vi "EnFlo_Data_Sync_Manual.vi"() -> ()   [LabVIEW 2012]
uses:
  Anemometry Sub Vis/Controls/EnFlo_Data_Folder_Setup.ctl
  Anemometry Sub Vis/Globals/Preference_global.vi
  Anemometry Sub Vis/Globals/Constants_global.vi
panel:
  out "error out":errorcluster
  out "Folder contents changed?":bool
  in  "Folder to Sync (Must be within Local EnFlo Data)":path=path "C:/EnFlo_Data_Temp/EnFlo_Software_SVN"
  in  "Get all Server Files":bool
  in  "Check Updates on Server?":bool
  in  "Archive Files?":bool
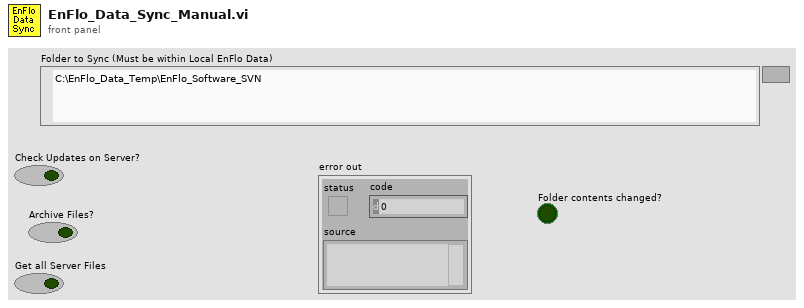
[diagram p1: front panel]
types:
  T1 = typedef "EnFlo_Data_Folder_Setup.ctl" = string
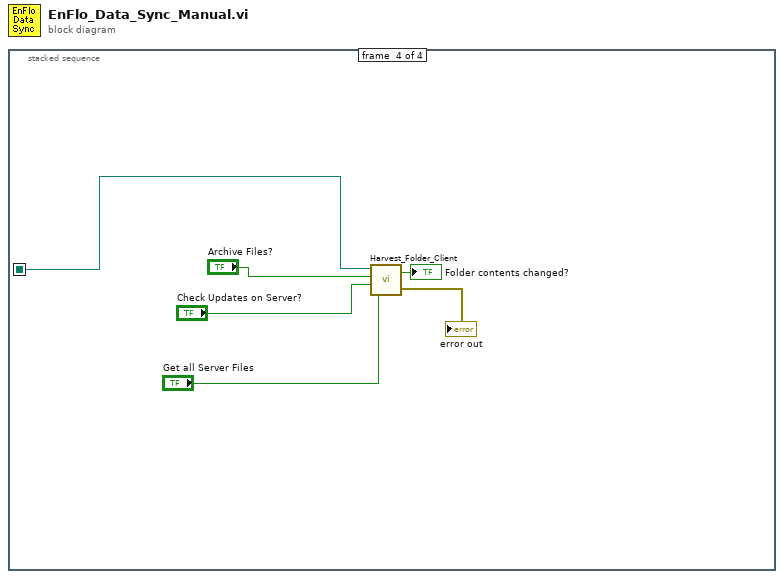
[diagram p0: block diagram]
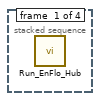
[diagram p2: hidden frame]
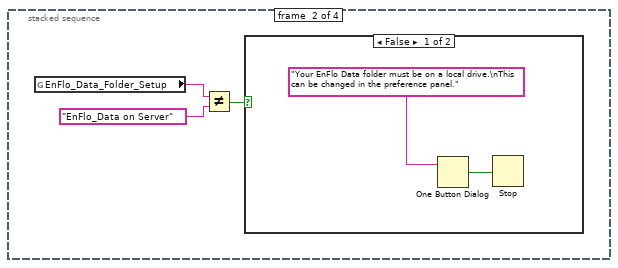
[diagram p3: hidden frame]
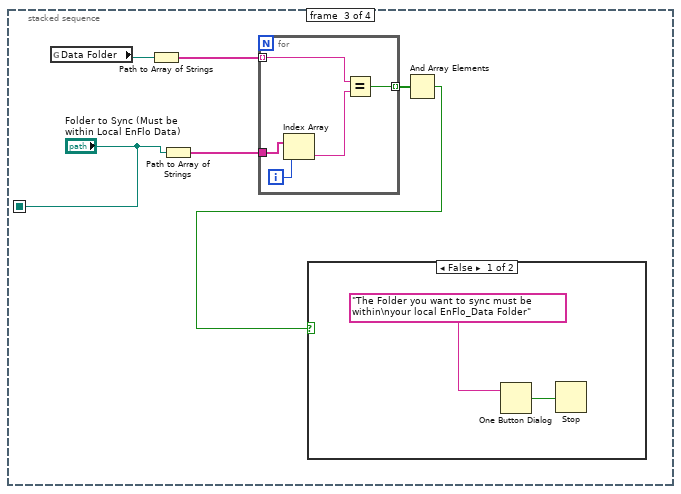
[diagram p5: hidden frame]
diagram:
  n1 = stacked-sequence {
    seq-local: [_ _ "Folder to Sync (Must be within Local EnFlo Data)" _] -> [_ _ _ w19]
    frame #0 {
      n2 = call "Run_EnFlo_Hub.vi"() -> ()  [unwired: 8 in]
    }
    frame #1 {
      n3 = global read "Preference_global.vi" "EnFlo_Data_Folder_Setup"() -> (w2:T1)
      n4 = Not Equal?(x=w2, y=T1 "EnFlo_Data on Server" ("EnFlo_Data_Folder_Setup")) -> (x != y?=w3:bool)
      n5 = case shown="False" w3 {
        frame False {
          n6 = One Button Dialog(message="Your EnFlo Data folder must be on a local drive.\nThis can be changed in the preference panel.") -> (true=w4:bool)  [unwired: 1 in]
          n7 = Stop(stop? (T)=w4) -> ()
        }
        frame True {
        }
      }
    }
    frame #2 {
      n8 = global read "Constants_global.vi" "Data Folder"() -> (w11:path)
      n9 = Path to Array of Strings(0:w11) -> (2:w9:string[])  [unwired: 1 out]
      n10 = Path to Array of Strings(0:"Folder to Sync (Must be within Local EnFlo Data)") -> (2:w10:string[])  [unwired: 1 out]
      n11 = for {
        tunnel: w10 -> [w16]
        tunnel: w9 -> [w14] mode=indexing
        tunnel: [w12] -> w8 mode=indexing
        i -> [w15]
        n12 = Index Array(array=w16, index=w15) -> (element=w13:string)
        n13 = Equal?(x=w14, y=w13) -> (x = y?=w12:bool)
      }
      n14 = And Array Elements(Boolean array=w8) -> (logical AND=w7:bool)
      n15 = case shown="False" w7 {
        frame False {
          n16 = One Button Dialog(message="The Folder you want to sync must be within\nyour local EnFlo_Data Folder") -> (true=w17:bool)  [unwired: 1 in]
          n17 = Stop(stop? (T)=w17) -> ()
        }
        frame True {
        }
      }
    }
    frame #3 {
      n18 = call "Harvest_Folder_Client.vi"("Get all Server Files"="Get all Server Files", "Check Updates on Server?"="Check Updates on Server?", "Archive Files?"="Archive Files?", "Folder to Harvest"=w19) -> ("error out"=→"error out":errorcluster, "Folder contents changed?"=→"Folder contents changed?":bool)
    }
  }
